vi "Config ODX Path.vi"(8 "error in (no error)":errorcluster, 11 "Parttype":T1) -> (0 "error out":errorcluster)   [LabVIEW 2018]
uses:
  typedefs/parttype.ctl
  <vilib>/Utility/config.llb/Read Key (Path).vi
  <vilib>/Utility/config.llb/Write Key (Path).vi
  <vilib>/Utility/config.llb/NI_LVConfig.lvlib
panel:
  in  "Cancel":bool
  out "Current Path":path
  in  "Save":bool
  in  "New Path":path
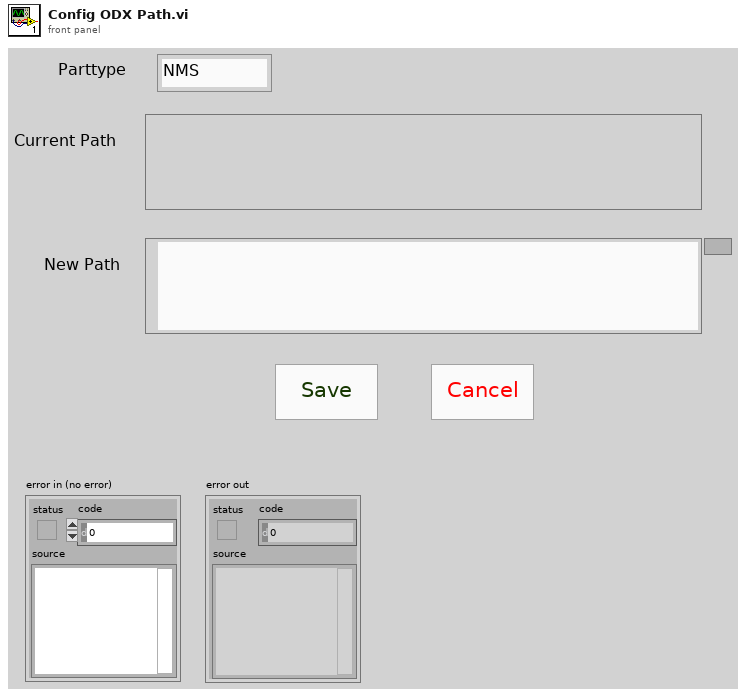
[diagram p1: front panel]
types:
  T1 = typedef "parttype.ctl" = enum16{"NMS", "B-SUV"}
  T2 = typedef "NI_LVConfig.lvlib/Config Data RefNum.ctl" = refnum<k1>
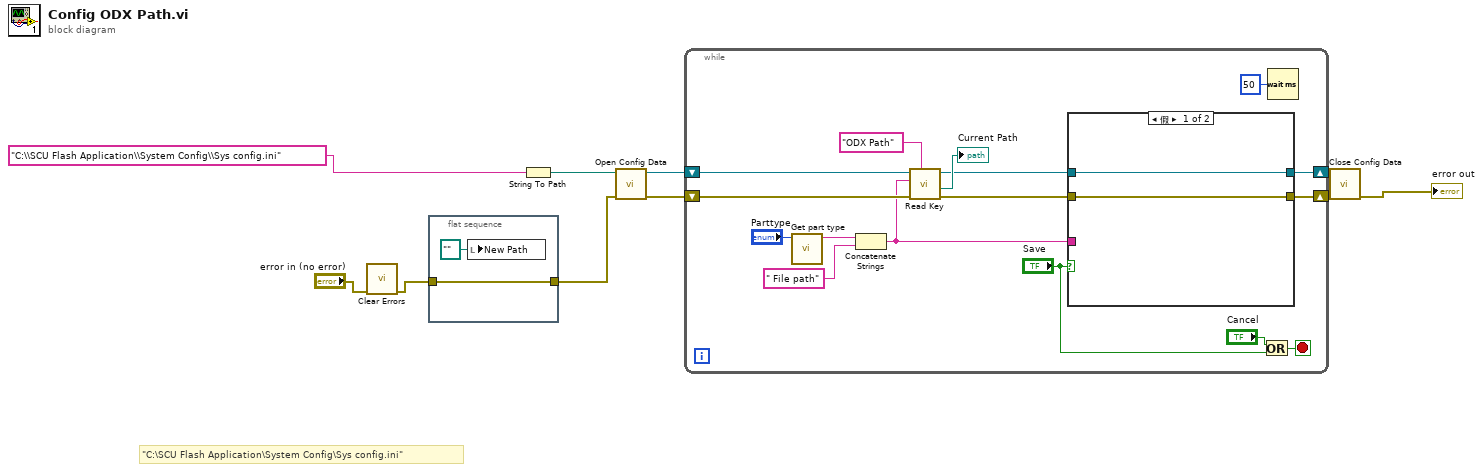
[diagram p0: block diagram]
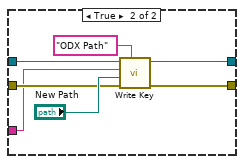
[diagram p2: hidden frame]
diagram:
  # "\"C:\\SCU Flash Application\\System Config\\Sys config.ini\""
  n1 = call <vilib>:"Clear Errors.vi"("error in (no error)"="error in (no error)") -> ("error out"=w2:errorcluster)  [unwired: 5 in, 1 out]
  n2 = flat-sequence {
    tunnel: w2 -> [w11]
    tunnel: [w11] -> w7
    frame #0 {
      n3 = local write "New Path"(path "" ("New Path")) -> ()
    }
  }
  n4 = String To Path(string="C:\\SCU Flash Application\\System Config\\Sys config.ini" ("name or relative path")) -> (path=w10:path)
  n5 = call <vilib>:"Open Config Data.vi"("error in (no error)"=w7, "configuration file path"=w10) -> ("error out"=w5:errorcluster, "refnum"=w6:T2)  [unwired: 7 in, 1 out]
  n6 = while {
    shift-right: [w27] -> w9
    shift-left: w6 -> [w17]
    shift-right: [w26] -> w8
    shift-left: w5 -> [w16]
    stop <- w25 stop-if-true
    n7 = call "Get part type.vi"("Enum"="Parttype") -> ("Parttype"=w20:string)  [unwired: 10 in]
    n8 = Concatenate Strings(w20, " File path" ("string")) -> (w13:string)
    n9 = call-poly <vilib>:"Read Key.vi"("section"="ODX Path", "error in (no error)"=w16, "key"=w13, "refnum"=w17) -> ("error out"=w15:errorcluster, "value"=→"Current Path":path, "refnum out"=w14:T2)  [unwired: 4 in, 1 out]
    n10 = case shown="假" "Save" {
      tunnel: w14 -> [w30 w37]
      tunnel: [w30 w34] -> w27
      tunnel: [w29 w33] -> w26
      tunnel: w15 -> [w29 w32]
      tunnel: w13 -> [_ w31]
      frame False {
      }
      frame True {
        n11 = call-poly <vilib>:"Write Key.vi"("section"="ODX Path", "error in (no error)"=w32, "value"="New Path", "key"=w31, "refnum"=w37) -> ("error out"=w33:errorcluster, "refnum out"=w34:T2)  [unwired: 4 in, 1 out]
      }
    }
    n12 = Or(x="Cancel", y="Save") -> (x .or. y?=w25:bool)
    n13 = Wait (ms)(milliseconds to wait=u32 50) -> ()  [unwired: 1 out]
  }
  n14 = call <vilib>:"Close Config Data.vi"("error in (no error)"=w8, "refnum"=w9) -> ("error out"=→"error out":errorcluster)  [unwired: 8 in, 1 out]
